vi "CreateVIPictures.vi"(8 "error in (no error)":errorcluster, 9 "Capture Target":T3=enum."Front Panel", 10 "VI 1 Screenshots":T1, 11 "Picture Save Location":path) -> (0 "error out":errorcluster, 2 "Screenshot Files":path[](array[path]))   [LabVIEW 2020, in "VIDiffScreenshots.lvlib"]
doc: "Captures .png imgaes of the VI given the path and the picture configuration."
uses:
  VIDiffScreenshots.lvlib
  Screenshot Type.ctl
  VIScreenshots.ctl
  ScreenshotInfo.ctl
  Utilities/FilePaths.ctl
  Utilities/VIDiffUtilities.lvlib
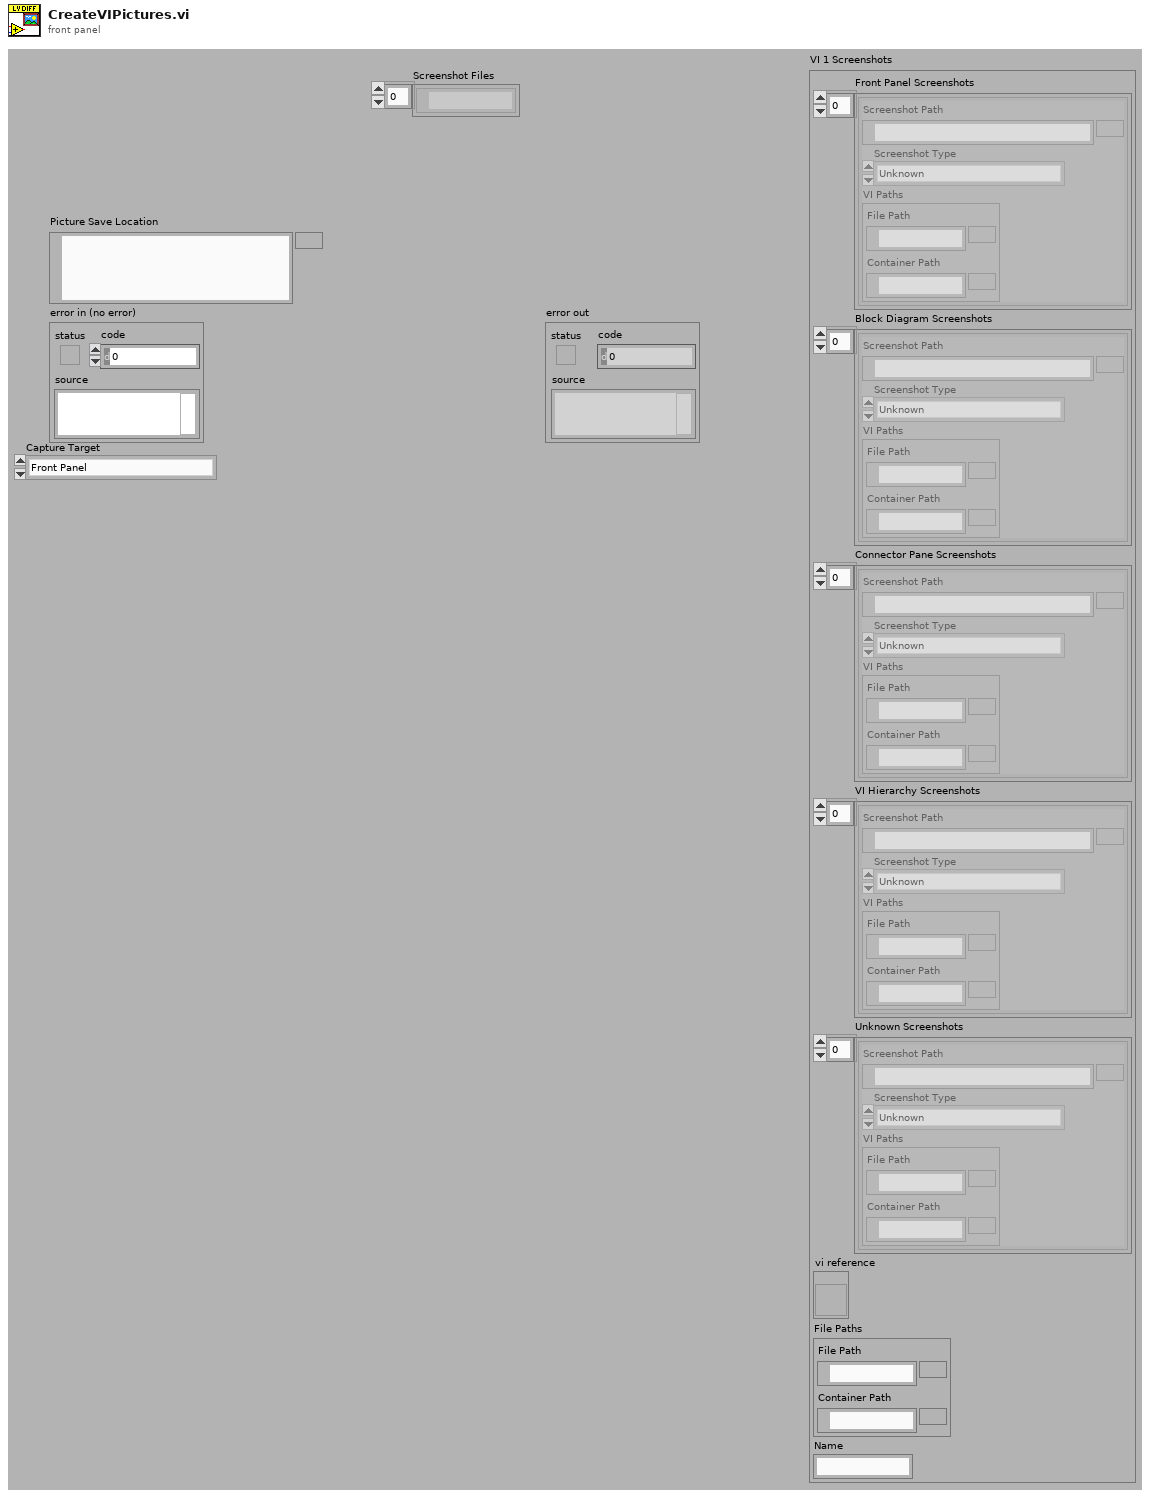
[diagram p1: front panel]
types:
  T1 = typedef "VIDiffScreenshots.lvlib/VIScreenshots.ctl" = cluster{"Front Panel Screenshots":T2[], "Block Diagram Screenshots":T2[], "Connector Pane Screenshots":T2[], "VI Hierarchy Screenshots":T2[], "Unknown Screenshots":T2[], "vi reference":refnum<vi>, "File Paths":cluster{"File Path":path, "Container Path":path}, "Name":string}
  T2 = typedef "VIDiffScreenshots.lvlib/ScreenshotInfo.ctl" = cluster{"Screenshot Path":path, "Screenshot Type":T3, "VI Paths":T4}
  T3 = typedef "VIDiffScreenshots.lvlib/Screenshot Type.ctl" = enum16{"Unknown", "Front Panel", "Connector Pane", "Block Diagram", "VI Hierarchy"}
  T4 = typedef "VIDiffUtilities.lvlib/FilePaths.ctl" = cluster{"File Path":path, "Container Path":path}
  T5 = cluster{"Printing:Custom All Controls?":bool, "Printing:Custom Connector?":bool, "Printing:Custom Control Descriptions?":bool, "Printing:Custom Control Types?":bool, "Printing:Custom Controls?":bool, "Printing:Custom Description?":bool, "Printing:Custom Diagram Hidden?":bool, "Printing:Custom Diagram Repeat?":bool, "Printing:Custom Diagram?":bool, "Printing:Custom Hierarchy?":bool, "Printing:Custom History?":bool, "Printing:Custom Panel Border?":bool, "Printing:Custom Panel?":bool, "Printing:Custom SubVIs?":bool}
  T6 = enum32{"Custom", "Standard", "Using Panel", "Using SubVI", "Complete"}
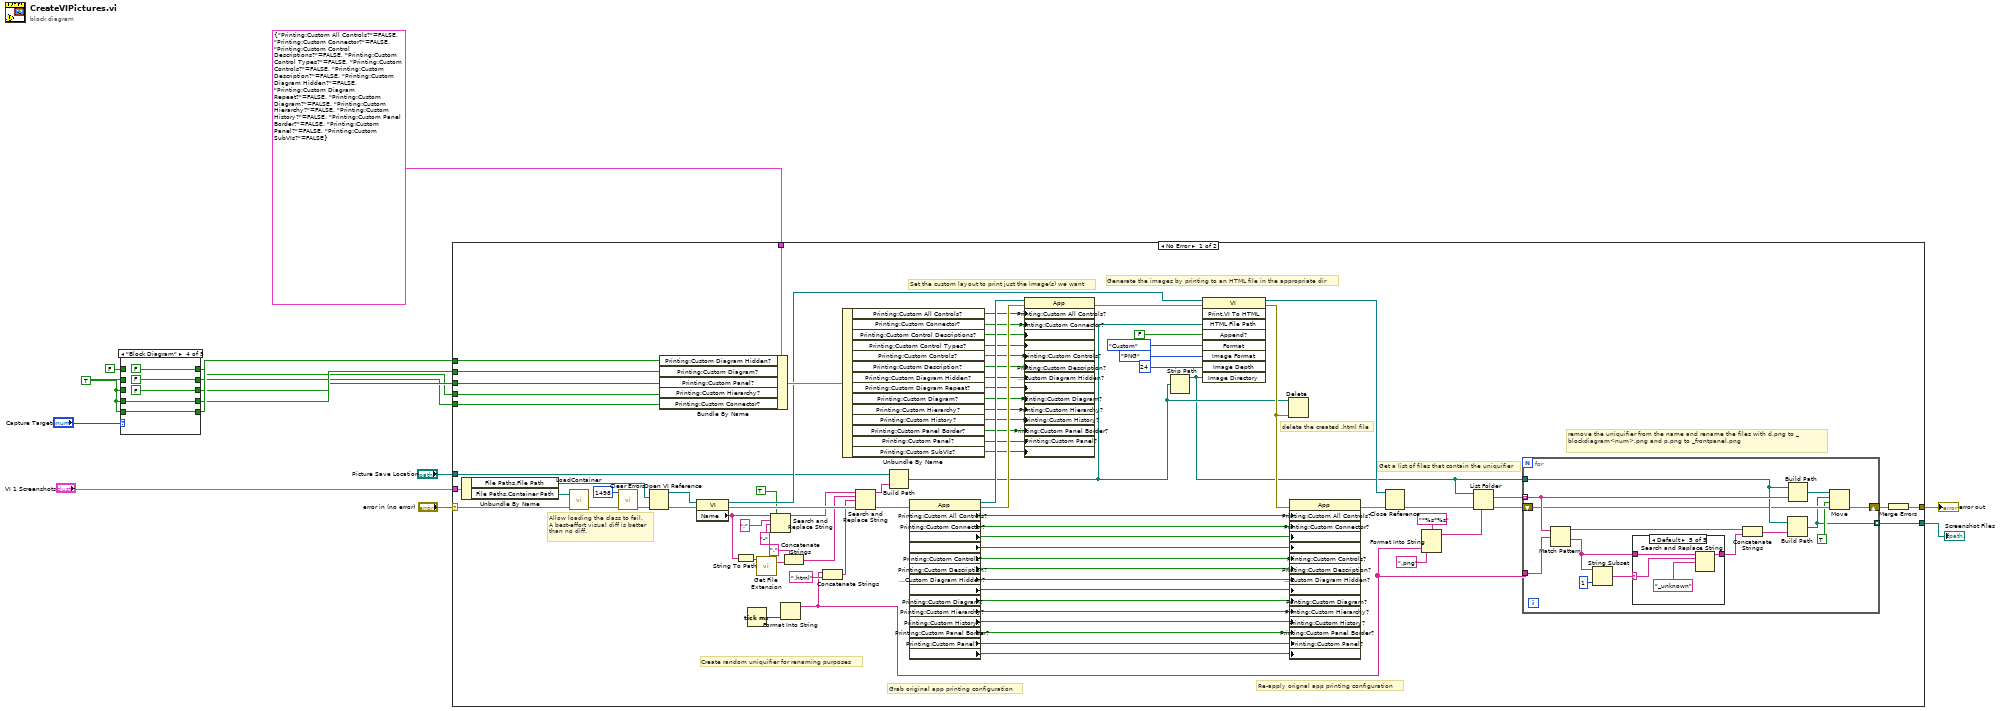
[diagram p0: block diagram]
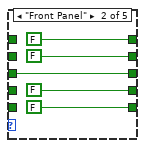
[diagram p3: hidden frame]
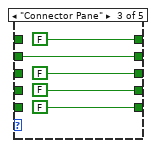
[diagram p4: hidden frame]
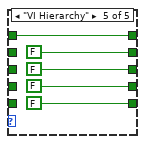
[diagram p5: hidden frame]
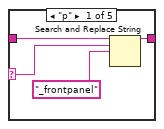
[diagram p6: hidden frame]
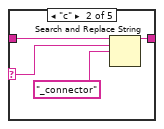
[diagram p7: hidden frame]
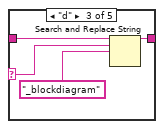
[diagram p8: hidden frame]
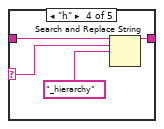
[diagram p9: hidden frame]
diagram:
  w6 = TRUE ("Capture Hierarchy?")
  n1 = case shown="\"Block Diagram\"" "Capture Target" {
    tunnel: FALSE ("Capture Hierarchy?") -> [w19 _ _ _ w35]
    tunnel: w6 -> [w18 _ w28 _ _]
    tunnel: w6 -> [w17 w24 _ _ _]
    tunnel: w6 -> [w16 _ _ w31 _]
    tunnel: w6 -> [w15 _ _ w30 _]
    tunnel: [w19 FALSE ("Capture Hierarchy?") FALSE ("Capture Hierarchy?") FALSE ("Capture Hierarchy?") w35] -> w2
    tunnel: [w18 FALSE ("Capture Connector?") w28 FALSE ("Capture Block Diagram?") FALSE ("Capture Block Diagram?")] -> w1
    tunnel: [w17 w24 FALSE ("Capture Block Diagram?") FALSE ("Capture Block Diagram?") FALSE ("Capture Block Diagram?")] -> w3
    tunnel: [w16 FALSE ("Capture Block Diagram?") FALSE ("Capture Block Diagram?") w31 FALSE ("Capture Block Diagram?")] -> w4
    tunnel: [w15 FALSE ("Capture Hidden Cases?") FALSE ("Capture Hidden Cases?") w30 FALSE ("Capture Block Diagram?")] -> w5
    frame "Unknown", Default {
    }
    frame "Front Panel" {
    }
    frame "Connector Pane" {
    }
    frame "Block Diagram" {
    }
    frame "VI Hierarchy" {
    }
  }
  n2 = case shown="No Error" "error in (no error)" {
    selector: "error in (no error)" -> [w46 w157]
    tunnel: T5 {"Printing:Custom All Controls?"=FALSE, "Printing:Custom Connector?"=FALSE, "Printing:Custom Control Descriptions?"=FALSE, "Printing:Custom Control Types?"=FALSE, "Printing:Custom Controls?"=FALSE, "Printing:Custom Description?"=FALSE, "Printing:Custom Diagram Hidden?"=FALSE, "Printing:Custom Diagram Repeat?"=FALSE, "Printing:Custom Diagram?"=FALSE, "Printing:Custom Hierarchy?"=FALSE, "Printing:Custom History?"=FALSE, "Printing:Custom Panel Border?"=FALSE, "Printing:Custom Panel?"=FALSE, "Printing:Custom SubVIs?"=FALSE} ("Content Options") -> [w122 _]
    tunnel: w5 -> [w121 _]
    tunnel: w4 -> [w120 _]
    tunnel: w3 -> [w119 _]
    tunnel: "Picture Save Location" -> [w78 _]
    tunnel: [w64 w157] -> w12
    tunnel: w2 -> [w63 _]
    tunnel: w1 -> [w62 _]
    tunnel: "VI 1 Screenshots" -> [w49 _]
    tunnel: [w43 _] -> w10
    frame No Error {
      # "Allow loading the class to fail.\nA best-effort visual diff is better\nthan no diff."
      # "remove the uniquifier from the name and rename the files with d.png to _blockdiagram<num>.png and p.png to _frontpanel.png"
      # "Get a list of files that contain the uniquifier"
      # "delete the created .html file"
      # "Create random uniquifier for renaming purposes"
      # "Re-apply orignal app printing configuration"
      # "Grab original app printing configuration"
      # "Generate the images by printing to an HTML file in the appropriate dir"
      # "Set the custom layout to print just the image(s) we want"
      n3 = Unbundle By Name(w49) -> ("File Paths.File Path"=w48:path, "File Paths.Container Path"=w47:path)
      n4 = call "LoadContainer.vi"("error in (no error)"=w46, "Container Path"=w47) -> ("error out"=w45:errorcluster)  [unwired: 9 in]
      n5 = call <vilib>:"Clear Errors.vi"("error in (no error)"=w45, "specific error code to clear (0: all)"=1498) -> ("error out"=w41:errorcluster)  [unwired: 4 in, 1 out]
      n6 = Open VI Reference(vi path=w48, error in (no error)=w41) -> (vi reference=w81:refnum<vi>, error out=w79:errorcluster)  [unwired: 4 in]
      n7 = Bundle By Name(cluster=w122, "Printing:Custom Diagram Hidden?"=w121, "Printing:Custom Diagram?"=w120, "Printing:Custom Panel?"=w119, "Printing:Custom Hierarchy?"=w63, "Printing:Custom Connector?"=w62) -> (w85:T5)
      n8 = property class="VI"(reference=w81, error in=w79) -> (reference out=w80:refnum<vi>, error out=w73:errorcluster, "Name"=w57:string)
      n9 = String To Path(string=w57) -> (path=w61:path)
      n10 = Tick Count (ms)() -> (millisecond timer value=w44:u32)
      n11 = call <vilib>:"Get File Extension.vi"("file"=w61) -> ("lowercase file extension"=w60:string)  [unwired: 6 in, 4 out]
      n12 = Search and Replace String(replace all?=TRUE ("replace all? (F)"), input string=w57, search string=":", replace string="-" ("replace string (\"\")")) -> (result string=w56:string)  [unwired: 4 in, 3 out]
      n13 = Format Into String(w44) -> (resulting string=w53:string)  [unwired: 3 in, 1 out]
      n14 = Concatenate Strings("." ("string"), w60) -> (w58:string)
      n15 = Concatenate Strings(w53, ".html" ("regular expression")) -> (w52:string)
      n16 = Unbundle By Name(w85) -> ("Printing:Custom All Controls?"=w99:bool, "Printing:Custom Connector?"=w98:bool, "Printing:Custom Control Descriptions?"=w97:bool, "Printing:Custom Control Types?"=w96:bool, "Printing:Custom Controls?"=w95:bool, "Printing:Custom Description?"=w94:bool, "Printing:Custom Diagram Hidden?"=w93:bool, "Printing:Custom Diagram Repeat?"=w92:bool, "Printing:Custom Diagram?"=w91:bool, "Printing:Custom Hierarchy?"=w90:bool, "Printing:Custom History?"=w89:bool, "Printing:Custom Panel Border?"=w88:bool, "Printing:Custom Panel?"=w87:bool, "Printing:Custom SubVIs?"=w86:bool)
      n17 = Search and Replace String(input string=w56, search string=w58, replace string=w52, error in=w73) -> (result string=w74:string, error out=w72:errorcluster)  [unwired: 4 in, 2 out]
      n18 = Build Path(base path=w78, name or relative path=w74) -> (appended path=w75:path)
      n19 = property class="App"(error in=w72) -> (reference out=w104:refnum<vi>, error out=w103:errorcluster, "Printing:Custom All Controls?"=w105:bool, "Printing:Custom Connector?"=w106:bool, "Printing:Custom Control Descriptions?"=w107:bool, "Printing:Custom Control Types?"=w108:bool, "Printing:Custom Controls?"=w109:bool, "Printing:Custom Description?"=w110:bool, "Printing:Custom Diagram Hidden?"=w111:bool, "Printing:Custom Diagram Repeat?"=w112:bool, "Printing:Custom Diagram?"=w113:bool, "Printing:Custom Hierarchy?"=w114:bool, "Printing:Custom History?"=w115:bool, "Printing:Custom Panel Border?"=w116:bool, "Printing:Custom Panel?"=w117:bool, "Printing:Custom List of SubVIs?"=w118:bool)  [unwired: 1 in]
      n20 = property class="App"(reference=w104, error in=w103, "Printing:Custom All Controls?"=w99, "Printing:Custom Connector?"=w98, "Printing:Custom Control Descriptions?"=w97, "Printing:Custom Control Types?"=w96, "Printing:Custom Controls?"=w95, "Printing:Custom Description?"=w94, "Printing:Custom Diagram Hidden?"=w93, "Printing:Custom Diagram Repeat?"=w92, "Printing:Custom Diagram?"=w91, "Printing:Custom Hierarchy?"=w90, "Printing:Custom History?"=w89, "Printing:Custom Panel Border?"=w88, "Printing:Custom Panel?"=w87, "Printing:Custom List of SubVIs?"=w86) -> (error out=w102:errorcluster)  [unwired: 1 out]
      n21 = Strip Path(path=w75) -> (stripped path=w67:path)  [unwired: 1 out]
      n22 = invoke class="VI" method="Print.VI To HTML"(reference=w80, error in=w102, "HTML File Path"=w75, "Append?"=FALSE, "Format"=T6."Custom", "Image Format"=enum32{"PNG", "JPEG", "GIF"}."PNG" ("Image Format (jpeg)"), "Image Depth"=24, "Image Directory"=w67) -> (reference out=w76:refnum<vi>, error out=w82:errorcluster)  [unwired: 1 in, 7 out]
      n23 = Delete(path (use dialog)=w75, error in=w82) -> ()  [unwired: 3 in, 3 out]
      n24 = property class="App"(error in=w82, "Printing:Custom All Controls?"=w105, "Printing:Custom Connector?"=w106, "Printing:Custom Control Descriptions?"=w107, "Printing:Custom Control Types?"=w108, "Printing:Custom Controls?"=w109, "Printing:Custom Description?"=w110, "Printing:Custom Diagram Hidden?"=w111, "Printing:Custom Diagram Repeat?"=w112, "Printing:Custom Diagram?"=w113, "Printing:Custom Hierarchy?"=w114, "Printing:Custom History?"=w115, "Printing:Custom Panel Border?"=w116, "Printing:Custom Panel?"=w117, "Printing:Custom List of SubVIs?"=w118) -> (error out=w77:errorcluster)  [unwired: 1 in, 1 out]
      n25 = Close Reference(reference=w76, error in (no error)=w77) -> (error out=w70:errorcluster)
      n26 = Format Into String(format string="*%s*%s" ("Format String"), w53, ".png" ("input 2")) -> (resulting string=w69:string)  [unwired: 2 in, 1 out]
      n27 = List Folder(path=w67, pattern=w69, error in=w70) -> (filenames=w66:string[], error out=w65:errorcluster)  [unwired: 1 in, 2 out]
      n28 = for {
        tunnel: w67 -> [w129]
        tunnel: w66 -> [w130] mode=indexing
        tunnel: w53 -> [w127]
        shift-right: [w125] -> w55
        shift-left: w65 -> [w126]
        tunnel: [w123] -> w43 mode=indexing
        n29 = Match Pattern(string=w130, regular expression=w127) -> (before substring=w132:string, after substring=w134:string)  [unwired: 1 in, 2 out]
        n30 = String Subset(string=w134, length (rest)=1 ("length (rest)")) -> (substring=w135:string)  [unwired: 1 in]
        n31 = case shown="Default" w135 {
          selector: w135 -> [w139 w143 w147 w151 w155]
          tunnel: w134 -> [w140 w144 w148 w152 w156]
          tunnel: [w137 w141 w145 w149 w153] -> w133
          frame "p" {
            n32 = Search and Replace String(input string=w140, search string=w139, replace string="_frontpanel" ("replace string (\"\")")) -> (result string=w137:string)  [unwired: 5 in, 3 out]
          }
          frame "c" {
            n33 = Search and Replace String(input string=w144, search string=w143, replace string="_connector" ("replace string (\"\")")) -> (result string=w141:string)  [unwired: 5 in, 3 out]
          }
          frame "d" {
            n34 = Search and Replace String(input string=w148, search string=w147, replace string="_blockdiagram" ("replace string (\"\")")) -> (result string=w145:string)  [unwired: 5 in, 3 out]
          }
          frame "h" {
            n35 = Search and Replace String(input string=w152, search string=w151, replace string="_hierarchy" ("replace string (\"\")")) -> (result string=w149:string)  [unwired: 5 in, 3 out]
          }
          frame Default {
            n36 = Search and Replace String(input string=w156, search string=w155, replace string="_unknown" ("replace string (\"\")")) -> (result string=w153:string)  [unwired: 5 in, 3 out]
          }
        }
        n37 = Concatenate Strings(w132, w133) -> (w131:string)
        n38 = Build Path(base path=w129, name or relative path=w131) -> (appended path=w123:path)
        n39 = Build Path(base path=w129, name or relative path=w130) -> (appended path=w128:path)
        n40 = Move(source path=w128, error in=w126, 9:TRUE ("overwrite (F)"), 10:w123) -> (error out=w125:errorcluster)  [unwired: 1 in, 2 out]
      }
      n41 = Merge Errors(w55) -> (w64:errorcluster)
    }
    frame Error {
    }
  }
  "error out" <- w12
  "Screenshot Files" <- w10
